vi "PH_HamamatsuCamera.destructor.vi"(0 "i ref in":refnum<vi>, 5 "error in(no error)":errorcluster) -> (19 "error out":errorcluster)   [LabVIEW 2014, in "PH_HamamatsuCamera.lvlib"]
doc: "This is the destructor of a class.\n\nLicense Agreement for this software:\n\nCopyright (C)\nGesellschaft für Schwerionenforschung, GSI\nPlanckstr. 1\n64291 Darmstadt\nGermany\n\nContact: D.Beck@gsi.de \n\nThis program is free software; you can redistribute it and/or modify it under the terms of the \nGNU General Public License as published by the Free Software Foundation; either version 2 of \nthe license, or (at your option) any later version.\n\nThis program is distributed in the hope that it will be useful, but WITHOUT ANY WARRANTY; \nwithout even the implied warranty of MERCHANTABILITY or FITNESS FOR A PARTICULAR PURPOSE. See the GNU General License for more details (http://www.gnu.org).\n\nGesellschaft für Schwerionenforschung, GSI\nPlanckstr. 1, 64291 Darmstadt, Germany\nFor all questions and ideas contact: M.Richter@gsi.de, H.Brand@gsi.de or D.Beck@gsi.de.\nLast update: 16-JUN-2004"
uses:
  PH_HamamatsuCamera.lvlib
  PH_Cam_BaseClass/PH_Cam_BaseClass.lvlib
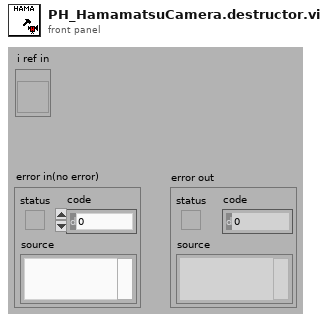
[diagram p1: front panel]
types:
  T1 = enum16{"SetAttribute", "GetAttribute", "CreateAttribute", "DestroyAttribute", "DestroyAllAtributes"}
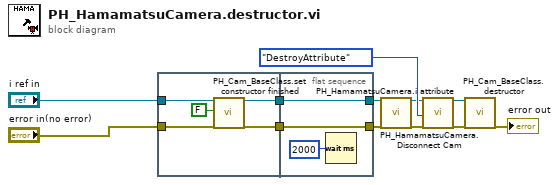
[diagram p0: block diagram]
diagram:
  n1 = flat-sequence {
    tunnel: "error in(no error)" -> [w16]
    tunnel: "i ref in" -> [w14]
    tunnel: [w15] -> w4
    tunnel: [w13] -> w3
    tunnel: [w19] -> w6
    tunnel: [w20] -> w8
    tunnel: w4 -> [w20]
    tunnel: w3 -> [w19]
    frame #0 {
      n2 = call "PH_Cam_BaseClass.set constructor finished.vi"("i ref in"=w14, "Contructor finished"=FALSE, "error in (no error)"=w16) -> ("i ref out"=w13:refnum<vi>, "error out"=w15:errorcluster)  [unwired: 15 in]
    }
    frame #1 {
      n3 = Wait (ms)(milliseconds to wait=u32 2000) -> ()  [unwired: 1 out]
    }
  }
  n4 = call "PH_HamamatsuCamera.Disconnect Cam.vi"("VI in"=w6, "error in (no error)"=w8) -> ("VI out"=w11:refnum<vi>, "error out"=w10:errorcluster)  [unwired: 16 in]
  n5 = call "PH_HamamatsuCamera.i attribute.vi"("VI Refnum"=w11, "Action"=T1."DestroyAttribute", "error in (no error)"=w10) -> ("VI Refnum out"=w2:refnum<vi>, "error out"=w5:errorcluster)  [unwired: 14 in, 1 out]
  n6 = call "PH_Cam_BaseClass.destructor.vi"("i ref in"=w2, "error in(no error)"=w5) -> ("error out"=→"error out":errorcluster)  [unwired: 17 in]
